vi "Send Vision Packet.vi"(7 "Camera":i16, 12 "Vision Targets":T2) -> ()   [LabVIEW 2013]
uses:
  Common Code/Goal Info.ctl
  Common Code/Vision Packet.ctl
  Common Code/Dashboard UDP/Omni Packet.ctl
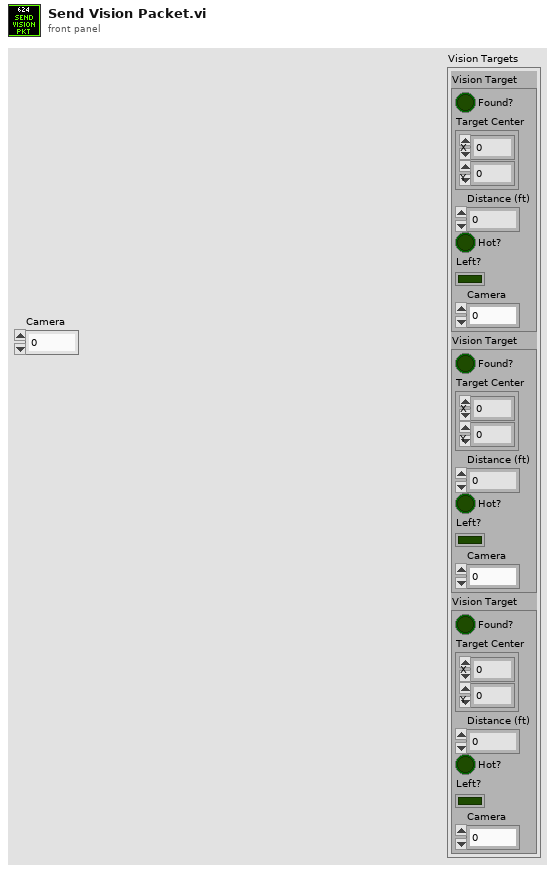
[diagram p1: front panel]
types:
  T1 = typedef "Goal Info.ctl" = cluster{"Found?":bool, "Target Center":cluster{"X":dbl, "Y":dbl}, "Distance (ft)":dbl, "Hot?":bool, "Left?":bool, "Camera":i16}
  T2 = cluster{"Vision Target":T1, "Vision Target":T1, "Vision Target":T1}
  T3 = typedef "Omni Packet.ctl" = cluster{"Type":i32, "data string":string}
  T4 = typedef "Vision Packet.ctl" = cluster{"Gyro":dbl, "Vision Target":T1, "Timestamp":u32, "Left Goal":T1, "Right Goal":T1}
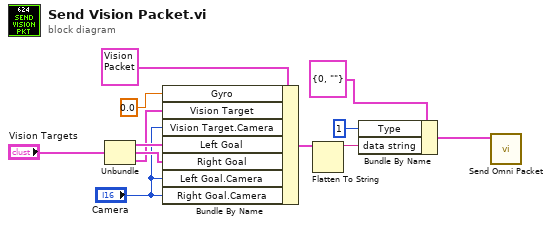
[diagram p0: block diagram]
diagram:
  n1 = Unbundle("Vision Targets") -> ("Vision Target"=w8:T1, "Vision Target"=w7:T1, "Vision Target"=w6:T1)
  n2 = Bundle By Name(cluster=T4 {"Gyro"=0.0, "Vision Target"={"Found?"=FALSE, "Target Center"={"X"=0.0, "Y"=0.0}, "Distance (ft)"=0.0, "Hot?"=FALSE, "Left?"=FALSE, "Camera"=0}, "Timestamp"=0, "Left Goal"={"Found?"=FALSE, "Target Center"={"X"=0.0, "Y"=0.0}, "Distance (ft)"=0.0, "Hot?"=FALSE, "Left?"=FALSE, "Camera"=0}, "Right Goal"={"Found?"=FALSE, "Target Center"={"X"=0.0, "Y"=0.0}, "Distance (ft)"=0.0, "Hot?"=FALSE, "Left?"=FALSE, "Camera"=0}} ("output cluster"), "Gyro"=0.0, "Vision Target"=w6, "Vision Target.Camera"="Camera", "Left Goal"=w8, "Right Goal"=w7, "Left Goal.Camera"="Camera", "Right Goal.Camera"="Camera") -> (w11:T4)
  n3 = Flatten To String(anything=w11) -> (data string=w2:string)  [unwired: 3 in, 2 out]
  n4 = Bundle By Name(cluster=T3 {"Type"=0, "data string"=""} ("OmniPacket"), "Type"=1, "data string"=w2) -> (w1:T3)
  n5 = call "Send Omni Packet.vi"("output cluster"=w1) -> ()  [unwired: 11 in]
